vi "Refresh Configuration.vi"(8 "error in (no error)":errorcluster, 11 "Configuration in":refnum<class "Configuration.lvclass">) -> (0 "error out":errorcluster, 3 "Configuration out":refnum<class "Configuration.lvclass">)   [LabVIEW 2023, in "Configuration.lvlib" / "Configuration.lvclass"]
doc: "Load configuration and signals list in to memory for reference.\nInspects the signal list for the defined device (if provided) and downselects the device's specific signal list."
uses:
  Library/Configuration.lvclass
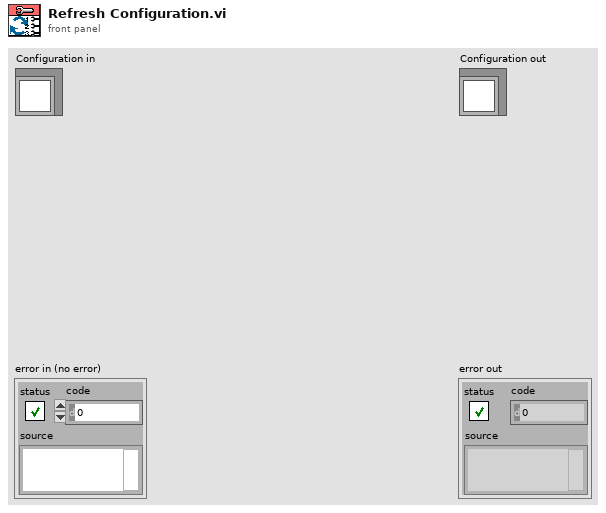
[diagram p1: front panel]
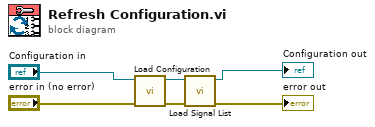
[diagram p0: block diagram]
diagram:
  n1 = call "Load Configuration.vi"("error in (no error)"="error in (no error)", "Configuration in"="Configuration in") -> ("error out"=w3:errorcluster, "Configuration out"=w4:refnum<class "Configuration.lvclass">)  [unwired: 8 in]
  n2 = call "Load Signal List.vi"("error in (no error)"=w3, "Configuration in"=w4) -> ("error out"=→"error out":errorcluster, "Configuration out"=→"Configuration out":refnum<class "Configuration.lvclass">)  [unwired: 8 in]
